vi "PID.vi"() -> ()   [LabVIEW 2019]
doc: "This example demonstrates how to simulate a general PID controller."
uses:
  <vilib>/addons/control/pid/pid.llb/PID (DBL).vi
  <vilib>/addons/control/pid/NI_PID_pid.lvlib
panel:
  out "Manipulated variable":dbl(graph)
  in  "SP:":dbl(slide)=43.790849673202615 min=0.0 max=0.0 scale=0.0..100.0
  out "MV:":dbl(slide)=18.78965245852964 scale=-100.0..100.0
  in  "PV:":dbl(slide)=60.754431603254424 scale=0.0..100.0
  in  "PID gains":T1={"proportional gain (Kc)"=20.0, "integral time (Ti, min)"=0.008, "derivative time (Td, min)"=0.001} {"derivative time (Td, min)" format="%.3f"; "integral time (Ti, min)" format="%.3f"; "proportional gain (Kc)" format="%.3f"}
  in  "Stop":bool
  out "Process variable and Setpoint":cluster{"initial PV":dbl, "SP:":dbl}(graph)
  # "Overview: This example demonstrates how to simulate a simple PID loop controller.\nInstructions:\n1. Run the VI and observe the Process variable (PV) following the Setpoint (SP) value while the output of the controller, also called Manipulated variable (MV), changes to keep both values near each other.\n2. After it settles down (value of PV and SP are near each other), change SP. You can just move the 'blue' arrow on the indicator. The MV will change to drive PV to SP again.\n3. Click Stop to stop the VI."
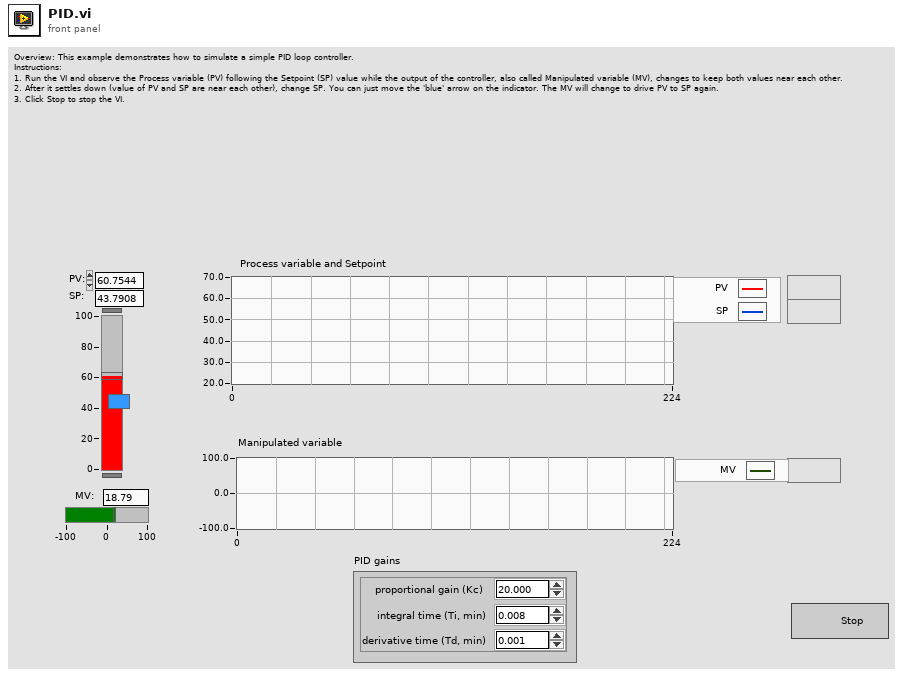
[diagram p1: front panel]
types:
  T1 = cluster{"proportional gain (Kc)":dbl, "integral time (Ti, min)":dbl, "derivative time (Td, min)":dbl}
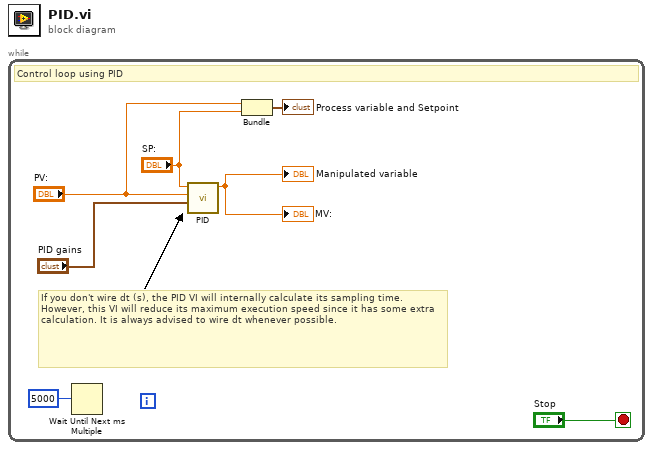
[diagram p0: block diagram]
diagram:
  n1 = while {
    stop <- "Stop" stop-if-true
    # "If you don't wire dt (s), the PID VI will internally calculate its sampling time. However, this VI will reduce its maximum execution speed since it has some extra calculation. It is always advised to wire dt whenever possible."
    # "Control loop using PID"
    n2 = Wait Until Next ms Multiple(millisecond multiple=u32 5000 ("unsigned 32bit integer")) -> ()  [unwired: 1 out]
    n3 = call-poly <vilib>:"PID.vi"("PID gains"="PID gains", "process variable"="PV:", "setpoint"="SP:") -> ("output"=→"MV:" →"Manipulated variable":dbl)  [unwired: 7 in, 1 out]
    n4 = Bundle("PV:"="PV:", "SP:"="SP:") -> (→"Process variable and Setpoint":cluster{"PV:":dbl, "SP:":dbl})  [unwired: 1 in]
  }
